vi "数据插入.vi"(5 "数据标记表":string(combo)="N", 7 "测量模式":string(combo), 8 "error in (no error)":errorcluster caption="错误输入（无错误）", 10 "data in":T1={"因子编码"="", "单位"="", "标样参考值"=0.0, "水样数据时间"=timestamp(0 s since 1904-01-01), "水样实测值"=0.0, "水样数据标识"="N", "探头温度"=0.0}, 11 "table输入":string(combo)) -> (0 "error out":errorcluster caption="错误输出")   [LabVIEW 2016, in "斯坦道多参数.lvlib"]
uses:
  <vilib>/Utility/sysdir.llb/System Directory Type.ctl
  <vilib>/Utility/error.llb/DialogType.ctl
  <vilib>/addons/database/Auxilliary.llb/DB Tools Transaction.ctl
  <vilib>/addons/database/Auxilliary.llb/DB Tools Isolation Level.ctl
  <vilib>/addons/database/Connection.llb/DB Tools Open Connec (String).vi
  <vilib>/addons/database/Connection.llb/Conn Execute.vi
  <vilib>/addons/database/Recordset.llb/Rec Destroy - Connection.vi
  <vilib>/addons/database/Connection.llb/Conn Transaction.vi
  <vilib>/addons/database/NI_Database_API.lvlib
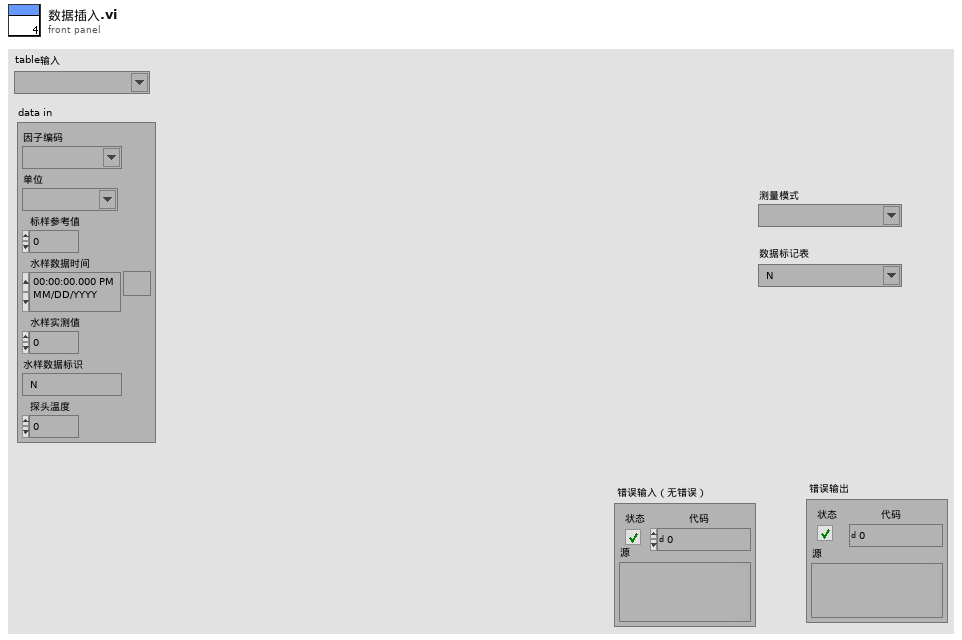
[diagram p1: front panel]
types:
  T1 = cluster{"因子编码":string, "单位":string, "标样参考值":sgl, "水样数据时间":timestamp, "水样实测值":sgl, "水样数据标识":string, "探头温度":sgl}
  T2 = typedef "NI_Database_API.lvlib/DB Tools Isolation Level.ctl" = enum16{"chaos", "read uncommitted", "read committed", "repeatable read", "serializable"}
  T3 = typedef "NI_Database_API.lvlib/DB Tools Transaction.ctl" = enum16{"begin", "commit", "rollback"}
  T4 = typedef "DialogType.ctl" = u16
  T5 = typedef "System Directory Type.ctl" = i32
  T6 = cluster{"时间标识":timestamp, "测量模式":string, "数据类型":string, "监测值":sgl, "单位":string, "数据标识":string, "因子编码":string, "标样参考值":sgl, "探头温度":sgl, "LastTime":timestamp}
  T7 = typedef "NI_Database_API.lvlib/Conn ObjectReference.ctl" = refnum<k1>
  T8 = typedef "NI_Database_API.lvlib/Rec ObjectReference.ctl" = refnum<k1>
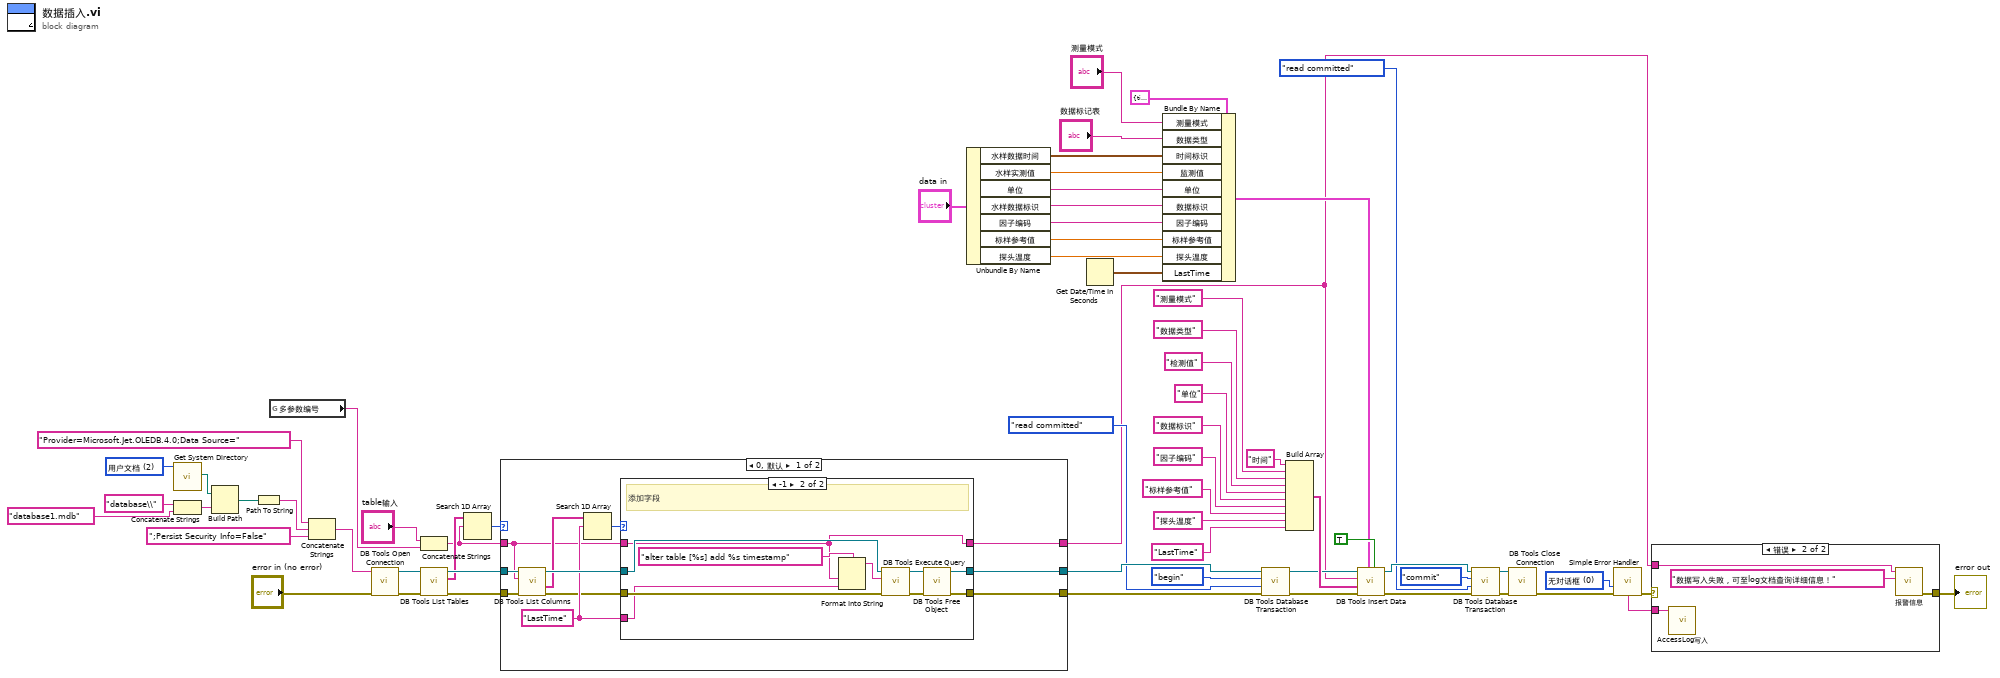
[diagram p0: block diagram]
diagram:
  w23 = T4 0 items=["无对话框", "确定信息", "继续或停止信息", "确定信息＋警告", "继续/停止+警告"] ("type of dialog (OK msg:1)")
  w45 = T5 2 items=["用户目录"=0, "用户桌面"=1, "用户文档"=2, "用户应用程序数据"=3, "用户设置"=4, "用户临时目录"=5, "公共文档"=6, "公共应用程序数据"=7, "公共设置"=8, "公共缓存"=13, "系统核心库"=9, "系统安装库"=10, "应用程序文件"=11, "启动盘根目录"=12] ("system directory type")
  n1 = call <vilib>:"Get System Directory.vi"("system directory type"=w45) -> ("system directory"=w43:path)  [unwired: 10 in]
  n2 = Concatenate Strings("database\\" ("condition"), "database1.mdb" ("字符串")) -> (w37:string)
  n3 = Build Path(base path=w43, name or relative path=w37) -> (appended path=w42:path)
  n4 = Path To String(path=w42) -> (string=w41:string)
  n5 = global read "多参数全局变量.vi" "多参数编号"() -> (w13:string)
  n6 = Concatenate Strings("Provider=Microsoft.Jet.OLEDB.4.0;Data Source=" ("condition"), w41, ";Persist Security Info=False" ("condition")) -> (w39:string)
  n7 = call-poly <vilib>:"DB Tools Open Connection.vi"("error in (no error)"="error in (no error)", "connection information"=w39) -> ("error out"=w12:errorcluster, "connection reference"=w29:T7)  [unwired: 6 in]
  n8 = Concatenate Strings("table输入", w13) -> (w14:string)
  n9 = call <vilib>:"DB Tools List Tables.vi"("error in (no error)"=w12, "connection reference"=w29) -> ("error out"=w18:errorcluster, "tables"=w17:string[], "connection reference out"=w19:T7)  [unwired: 3 in]
  n10 = Search 1D Array(1D array=w17, element=w14) -> (index of element=w15:i32)  [unwired: 1 in]
  n11 = case shown="0, 默认" w15 {
    tunnel: [w69 w90] -> w28
    tunnel: [w68 w88] -> w5
    tunnel: [w67 w89] -> w1
    tunnel: w19 -> [w66 w90]
    tunnel: w18 -> [w65 w88]
    tunnel: w14 -> [w64 w89]
    frame 0, Default {
      w73 = "LastTime" ("元素")
      n12 = call <vilib>:"DB Tools List Columns.vi"("error in (no error)"=w65, "table"=w64, "connection reference"=w66) -> ("error out"=w71:errorcluster, "columns"=w72:string[], "connection reference out"=w74:T7)  [unwired: 1 in, 1 out]
      n13 = Search 1D Array(1D array=w72, element=w73) -> (index of element=w70:i32)  [unwired: 1 in]
      n14 = case shown="-1" w70 {
        tunnel: w74 -> [w77 w85]
        tunnel: w71 -> [w76 w84]
        tunnel: w73 -> [_ w82]
        tunnel: [w77 w80] -> w69
        tunnel: [w76 w79] -> w68
        tunnel: w64 -> [w75 w78]
        tunnel: [w75 w78] -> w67
        frame 0, Default {
        }
        frame -1 {
          # "添加字段"
          n15 = Format Into String(format string="alter table [%s] add %s timestamp", w78, w82) -> (resulting string=w81:string)  [unwired: 2 in, 1 out]
          n16 = call-poly <vilib>:"DB Tools Execute Query.vi"("error in (no error)"=w84, "SQL query"=w81, "connection reference"=w85) -> ("error out"=w86:errorcluster, "recordset reference"=w87:T8)  [unwired: 5 in]
          n17 = call-poly <vilib>:"DB Tools Free Object.vi"("error in (no error)"=w86, "recordset reference"=w87) -> ("error out"=w79:errorcluster, "connection reference"=w80:T7)  [unwired: 8 in]
        }
      }
    }
    frame -1 {
    }
  }
  n18 = Unbundle By Name("data in") -> ("水样数据时间"=w58:timestamp, "水样实测值"=w57:sgl, "单位"=w53:string, "水样数据标识"=w56:string, "因子编码"=w52:string, "标样参考值"=w54:sgl, "探头温度"=w34:sgl)
  n19 = Get Date/Time In Seconds() -> (seconds since 1Jan1904=w26:timestamp)
  n20 = Bundle By Name(cluster=T6 {"时间标识"=timestamp(0 s since 1904-01-01), "测量模式"="", "数据类型"="", "监测值"=0.0, "单位"="", "数据标识"="", "因子编码"="", "标样参考值"=0.0, "探头温度"=0.0, "LastTime"=timestamp(0 s since 1904-01-01)} ("data输出"), "测量模式"="测量模式", "数据类型"="数据标记表", "时间标识"=w58, "监测值"=w57, "单位"=w53, "数据标识"=w56, "因子编码"=w52, "标样参考值"=w54, "探头温度"=w34, "LastTime"=w26) -> (w35:T6)
  n21 = call-poly <vilib>:"DB Tools Database Transaction.vi"("error in (no error)"=w5, "isolation level (chaos)"=DB_Tools_Isolation_Level."read committed", "operation (begin)"=DB_Tools_Transaction."begin", "connection reference"=w28) -> ("error out"=w3:errorcluster, "connection reference out"=w6:T7)  [unwired: 2 in]
  n22 = Build Array("时间", "测量模式", "数据类型", "检测值", "单位", "数据标识", "因子编码", "标样参考值", "探头温度", "LastTime") -> (w36:string[])
  n23 = call <vilib>:"DB Tools Insert Data.vi"("create table? (F)"=TRUE, "data"=w35, "error in (no error)"=w3, "columns"=w36, "table"=w1, "connection reference"=w6) -> ("error out"=w8:errorcluster, "connection reference out"=w47:T7)  [unwired: 4 in]
  n24 = call-poly <vilib>:"DB Tools Database Transaction.vi"("error in (no error)"=w8, "isolation level (chaos)"=DB_Tools_Isolation_Level."read committed", "operation (begin)"=DB_Tools_Transaction."commit", "connection reference"=w47) -> ("error out"=w7:errorcluster, "connection reference out"=w11:T7)  [unwired: 2 in]
  n25 = call <vilib>:"DB Tools Close Connection.vi"("error in (no error)"=w7, "connection reference"=w11) -> ("error out"=w24:errorcluster)  [unwired: 5 in]
  n26 = call <vilib>:"Simple Error Handler.vi"("type of dialog (OK msg:1)"=w23, "error in (no error)"=w24) -> ("error out"=w21:errorcluster, "message"=w22:string)  [unwired: 3 in, 3 out]
  n27 = case shown="错误" w21 {
    selector: w21 -> [w91 _]
    tunnel: w22 -> [_ w93]
    tunnel: [w91 w95] -> w20
    tunnel: w1 -> [_ w94]
    frame No Error {
    }
    frame Error {
      n28 = call "AccessLog写入.vi"("Log"=w93) -> ()  [unwired: 11 in]
      n29 = call "报警信息.vi"("报警信息"="数据写入失败，可至log文档查询详细信息！", "设备"=w94) -> ("error out"=w95:errorcluster)  [unwired: 9 in]
    }
  }
  "error out" <- w20
